vi "Write Double.vi"(7 "Channel Array in":refnum<class "CIFChannels.lvclass">[](array[class]), 8 "error in (no error)":errorcluster, 9 "Data":dbl, 10 "Channel Index":i32) -> (0 "error out":errorcluster, 1 "timed out?":bool, 5 "Channel Array out":refnum<class "CIFChannels.lvclass">[](array[class]))   [LabVIEW 2021, in "CIFChannelMng.lvclass"]
uses:
  CIFChannelMng.lvclass
  <vilib>/CIF Foundation/CIF Channels Core/CIFChannels/CIFChannels.lvclass
  CIFChannelMng.lvclass/CIFChannelMng.ctl
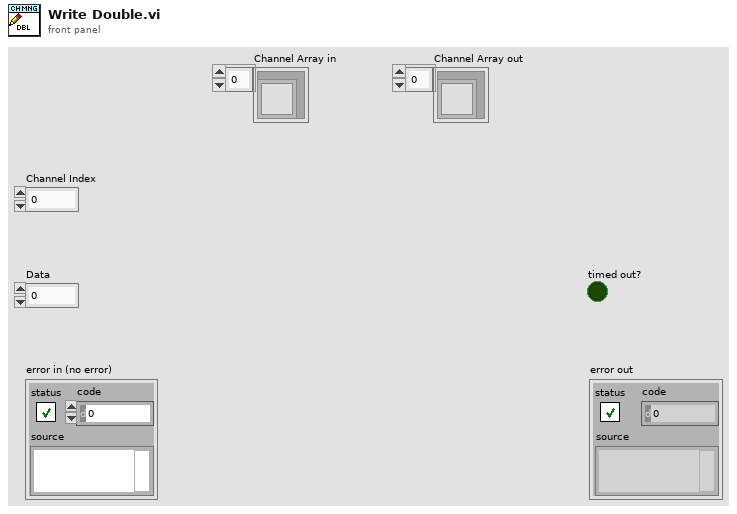
[diagram p1: front panel]
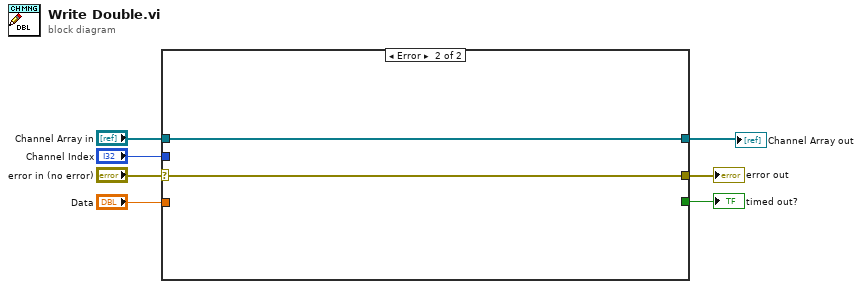
[diagram p0: block diagram]
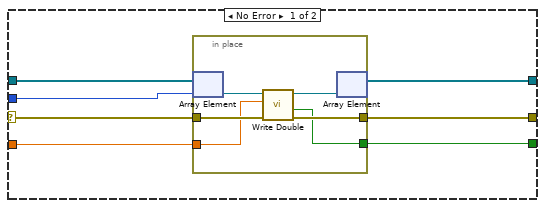
[diagram p2: hidden frame]
diagram:
  n1 = case shown="Error" "error in (no error)" {
    selector: "error in (no error)" -> [w14 w22]
    tunnel: [w13 w22] -> w6
    tunnel: "Channel Array in" -> [w8 w21]
    tunnel: "Data" -> [w12 _]
    tunnel: [w11 _] -> w4
    tunnel: "Channel Index" -> [w10 _]
    tunnel: [w9 w21] -> w1
    frame No Error {
      n2 = in-place {
        in-place-border: w14 -> [w20]
        in-place-border: [w19] -> w13
        in-place-border: [w18] -> w11
        in-place-border: w12 -> [w17]
        n3 = in-place-array #1(w8, w10) -> (w16:refnum<class "CIFChannels.lvclass">)
        n4 = call-dynamic "Write Double.vi"("error in (no error)"=w20, "Data"=w17, "CIFChannels in"=w16) -> ("error out"=w19:errorcluster, "timed out?"=w18:bool, "CIFChannels out"=w15:refnum<class "CIFChannels.lvclass">)  [unwired: 6 in]
        n5 = in-place-array #1(w15) -> (w9:refnum<class "CIFChannels.lvclass">[])  [unwired: 1 out]
      }
    }
    frame Error {
    }
  }
  "error out" <- w6
  "timed out?" <- w4
  "Channel Array out" <- w1
